vi "Startup.vi"(11 "Started":refnum<notifier>) -> ()   [LabVIEW 2024, in "Startup.lvlib"]
uses:
  Startup.lvlib
  States.ctl
  ModuleTemplates/ErrorHandler/ErrorHandler.lvclass
  ModuleTemplates/ModuleManager/ModuleManager.lvclass
  ModuleTemplates/UIManager/UIManager.lvclass
  RQMHCore/DebugTrace/FGVWithEventTrace/FGVWithEventTrace.lvclass
  RQMHCore/ModuleCore/RQMHModule.lvclass
  RQMHCore/DebugTrace/DebugTraceSingleton/DebugTraceSingleton.lvlib
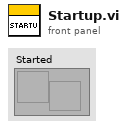
[diagram p1: front panel]
types:
  T1 = typedef "Startup.lvlib/States.ctl" = enum16{"Init", "StartCore", "StartModules", "Register", "Ready", "Wait", "Unregister", "StopModules", "StopCore", "Exit", "Error"}
  T2 = cluster{"ErrorManager":refnum<class "ErrorHandler.lvclass">, "ModuleManager":refnum<class "ModuleManager.lvclass">, "UIManager":refnum<class "UIManager.lvclass">}
  T3 = typedef "RQMHModule.lvclass/StandardBroadcasts.ctl" = cluster{"Died":refnum<user-event>, "Started":refnum<user-event>}
  T4 = typedef "UIManager.lvclass/Broadcast Events--cluster.ctl" = cluster{"Stopped":refnum<user-event>, "Request Stop":refnum<user-event>}
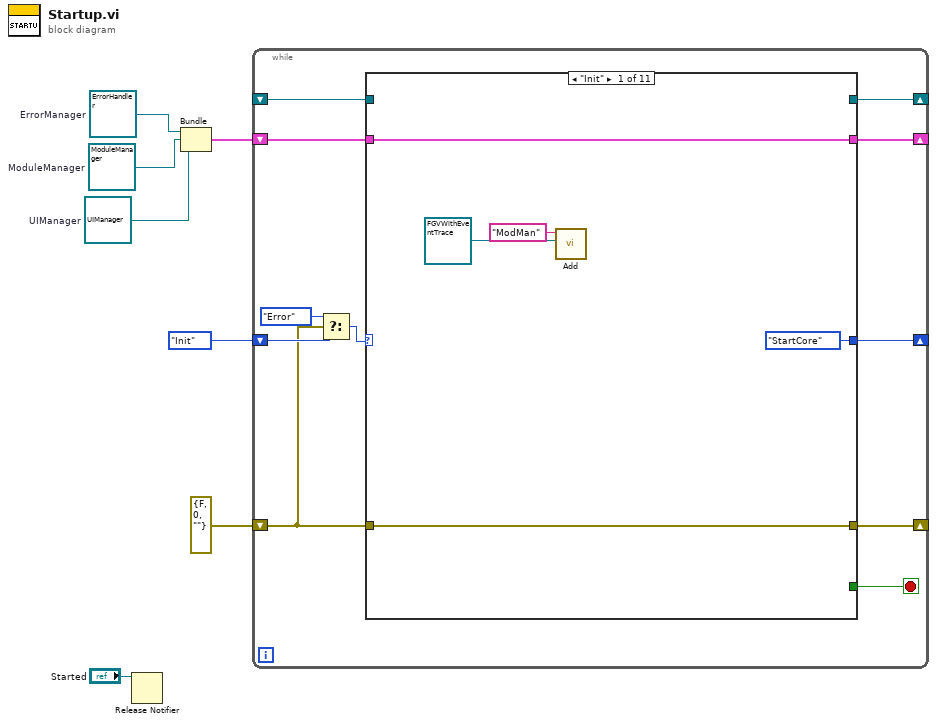
[diagram p0: block diagram]
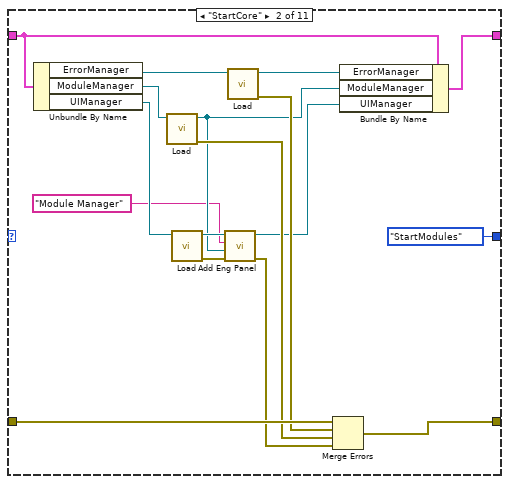
[diagram p2: hidden frame]
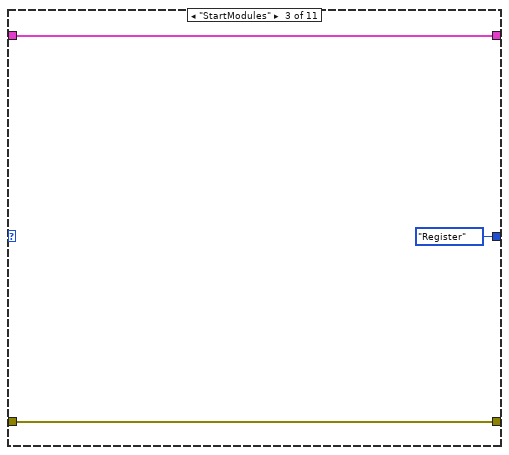
[diagram p3: hidden frame]
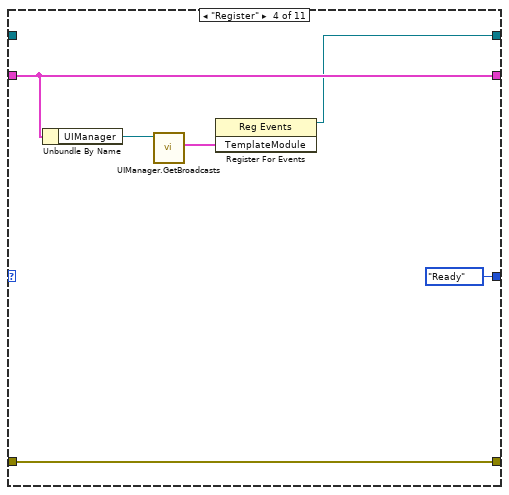
[diagram p4: hidden frame]
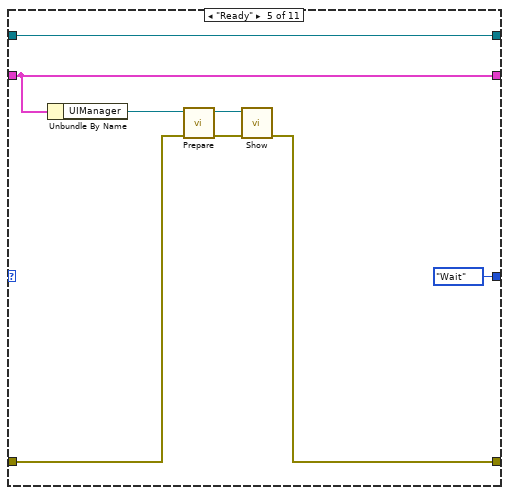
[diagram p5: hidden frame]
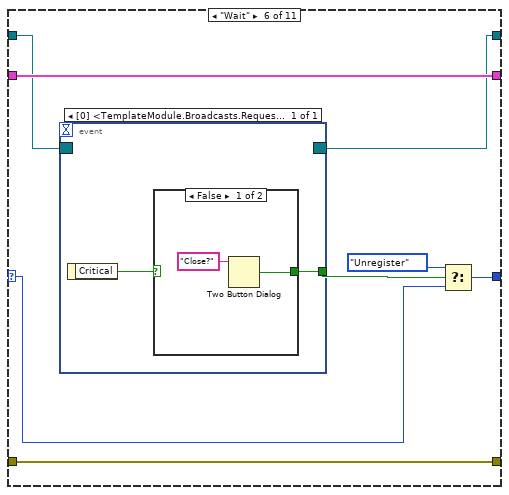
[diagram p6: hidden frame]
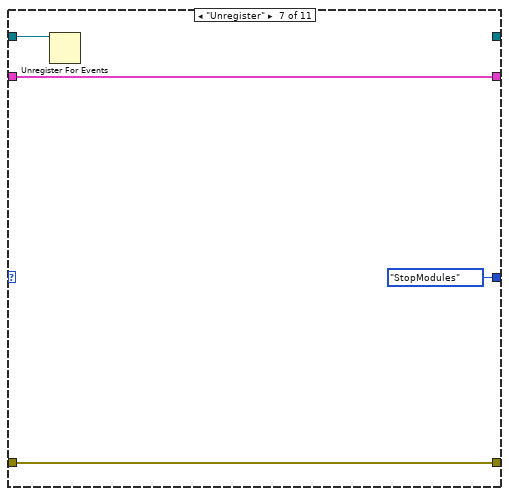
[diagram p8: hidden frame]
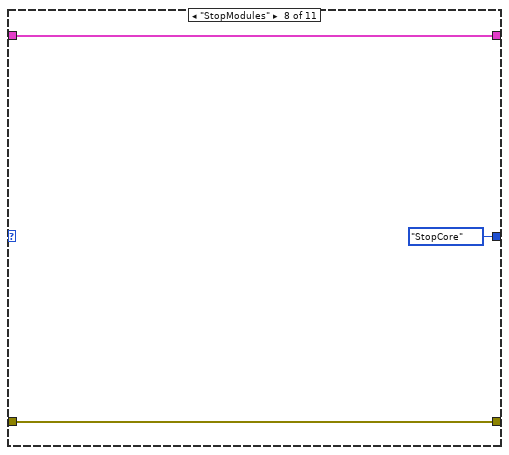
[diagram p9: hidden frame]
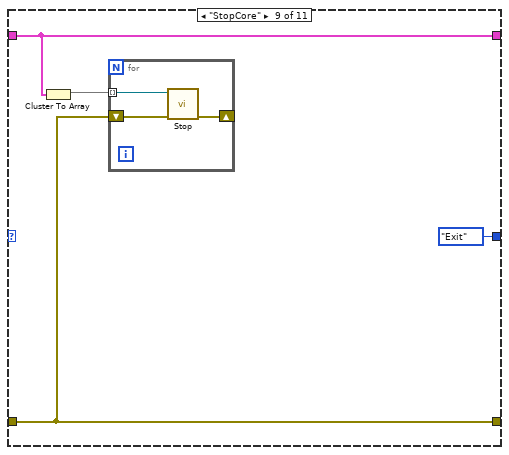
[diagram p10: hidden frame]
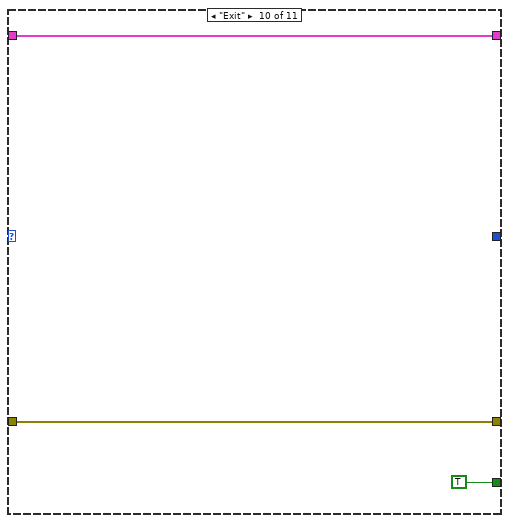
[diagram p11: hidden frame]
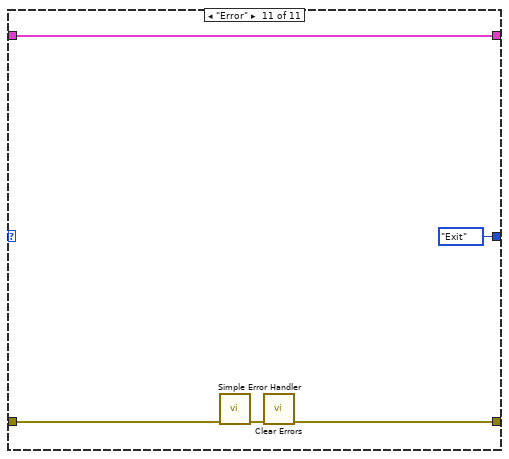
[diagram p12: hidden frame]
diagram:
  w1 = refnum<class "UIManager.lvclass"> refnum  # UIManager
  w2 = refnum<class "ModuleManager.lvclass"> refnum  # ModuleManager
  w3 = refnum<class "ErrorHandler.lvclass"> refnum  # ErrorManager
  n1 = Release Notifier(notifier="Started") -> ()  [unwired: 2 in, 3 out]
  n2 = Bundle("ErrorManager"=w3, "ModuleManager"=w2, "UIManager"=w1) -> (w4:T2)  [unwired: 1 in]
  n3 = while {
    shift-right: [w15] -> _
    shift-left: errorcluster {"status"=FALSE, "code"=0, "source"=""} ("error in (no error)") -> [w14]
    shift-right: [w11] -> _
    shift-left: States."Init" ("States") -> [w18]
    shift-right: [w12] -> _
    shift-left: w4 -> [w13]
    shift-right: [w10] -> _
    shift-left: _ -> [w9]
    stop <- w8 stop-if-true
    n4 = Select(t=States."Error" ("States"), s=w14, f=w18) -> (s? t:f=w16:T1)
    n5 = case shown="\"Init\"" w16 {
      selector: w16 -> [_ _ _ _ _ w61 _ _ _ _ _]
      tunnel: [w23 w33 w43 w49 w50 w65 w74 w77 w79 w87 w88] -> w15
      tunnel: w14 -> [w23 w40 w43 w49 w53 w65 w74 w77 w79 w87 w91]
      tunnel: w13 -> [w22 w29 w42 w46 w55 w64 w73 w76 w81 w86 w92]
      tunnel: [w22 w30 w42 w46 w55 w64 w73 w76 w81 w86 w92] -> w12
      tunnel: [States."StartCore" ("States") States."StartModules" ("States") States."Register" ("States") States."Ready" ("States") States."Wait" ("States") w62 States."StopModules" ("States") States."StopCore" ("States") States."Exit" ("States") _ States."Exit" ("States")] -> w11
      tunnel: [_ _ _ w44 w56 w58 _ _ _ _ _] -> w10
      tunnel: w9 -> [_ _ _ _ w56 w63 w72 _ _ _ _]
      tunnel: [_ _ _ _ _ _ _ _ _ TRUE _] -> w8
      frame "Init" {
        n6 = call "Add.vi"("DebugTracer"=refnum<class "FGVWithEventTrace.lvclass"> refnum ("FGVWithEventTrace.lvclass"), "Name"="ModMan") -> ()  [unwired: 10 in]
      }
      frame "StartCore" {
        n7 = Unbundle By Name(w29) -> ("ErrorManager"=w39:refnum<class "ErrorHandler.lvclass">, "ModuleManager"=w37:refnum<class "ModuleManager.lvclass">, "UIManager"=w36:refnum<class "UIManager.lvclass">)
        n8 = call "Load.vi"("RQMHModule in"=w37) -> ("error out"=w31:errorcluster, "RQMHModule out"=w27:refnum<class "ModuleManager.lvclass">)  [unwired: 9 in]
        n9 = call "Load.vi"("RQMHModule in"=w36) -> ("error out"=w25:errorcluster, "RQMHModule out"=w35:refnum<class "UIManager.lvclass">)  [unwired: 9 in]
        n10 = call "Add Eng Panel.vi"("error in (no error)"=w25, "EngPanel"=w27, "Name"="Module Manager", "module in"=w35) -> ("error out"=w24:errorcluster, "module out"=w28:refnum<class "UIManager.lvclass">)  [unwired: 5 in, 1 out]
        n11 = call "Load.vi"("RQMHModule in"=w39) -> ("error out"=w32:errorcluster, "RQMHModule out"=w38:refnum<class "ErrorHandler.lvclass">)  [unwired: 9 in]
        n12 = Merge Errors(w40, w32, w31, w24) -> (w33:errorcluster)
        n13 = Bundle By Name(cluster=w29, "ErrorManager"=w38, "ModuleManager"=w27, "UIManager"=w28) -> (w30:T2)
      }
      frame "StartModules" {
      }
      frame "Register" {
        n14 = Unbundle By Name(w46) -> ("UIManager"=w45:refnum<class "UIManager.lvclass">)
        n15 = call "UIManager.GetBroadcasts.vi"("NewTemplate in"=w45) -> ("TemplateModule"=w47:cluster{"Broadcasts":T3, "Broadcasts":T4})  [unwired: 9 in, 1 out]
        n16 = register-events(w47) -> (reference out=w44:refnum<event-registration>)  [unwired: 2 in, 1 out]
      }
      frame "Ready" {
        n17 = Unbundle By Name(w55) -> ("UIManager"=w54:refnum<class "UIManager.lvclass">)
        n18 = call "Prepare.vi"("error in (no error)"=w53, "module in"=w54) -> ("error out"=w51:errorcluster, "module out"=w52:refnum<class "UIManager.lvclass">)  [unwired: 6 in, 2 out]
        n19 = call "Show.vi"("error in (no error)"=w51, "module in"=w52) -> ("error out"=w50:errorcluster)  [unwired: 7 in, 2 out]
      }
      frame "Wait" {
        n20 = event shown="[0] <TemplateModule.Broadcasts.Request Stop>: User Event" {
          selector: w63 -> [_]
          dyn-events: [_] -> w58
          timeout: _ -> [_]
          tunnel: [w66] -> w60
          event User Event {
            n21 = event-data() -> ("Critical"=w67:bool)  [unwired: 1 in]
            n22 = case shown="False" w67 {
              selector: w67 -> [_ w70]
              tunnel: [w69 w70] -> w66
              frame False {
                n23 = Two Button Dialog(message="Close?") -> (T button?=w69:bool)  [unwired: 2 in]
              }
              frame True {
              }
            }
          }
        }
        n24 = Select(t=States."Unregister", s=w60, f=w61) -> (s? t:f=w62:T1)
      }
      frame "Unregister" {
        n25 = Unregister For Events(event registration refnum=w72) -> ()  [unwired: 1 in, 1 out]
      }
      frame "StopModules" {
      }
      frame "StopCore" {
        n26 = Cluster To Array(cluster=w81) -> (array=w80:refnum<class "RQMHModule.lvclass">[])
        n27 = for {
          tunnel: w80 -> [w84] mode=indexing
          shift-right: [w82] -> _
          shift-left: w79 -> [w83]
          n28 = call "Stop.vi"("error in (no error)"=w83, "JQMHCore in"=w84) -> ("error out"=w82:errorcluster)  [unwired: 9 in]
        }
      }
      frame "Exit" {
      }
      frame "Error" {
        n29 = call <vilib>:"Simple Error Handler.vi"("error in (no error)"=w91) -> ("error out"=w89:errorcluster)  [unwired: 4 in, 4 out]
        n30 = call <vilib>:"Clear Errors.vi"("error in (no error)"=w89) -> ("error out"=w88:errorcluster)  [unwired: 5 in, 1 out]
      }
    }
  }
